vi "Constructor.vi"(8 "error in (no error)":errorcluster, 10 "lines":tag, 11 "Solenoid Valve in":refnum<class "Solenoid Valve.lvclass">) -> (0 "error out":errorcluster, 3 "Solenoid Valve out":refnum<class "Solenoid Valve.lvclass">)   [LabVIEW 2011, in "Solenoid Valve.lvclass"]
uses:
  Solenoid Valve.lvclass
  Solenoid Valve.lvclass/Solenoid Valve.ctl
  <vilib>/DAQmx/write.llb/DAQmx Write (Digital Bool 1Line 1Point).vi
  <vilib>/DAQmx/create/channels.llb/DAQmx Create Channel (DO-Digital Output).vi
  <vilib>/DAQmx/miscellaneous.llb/DAQmx Fill In Error Info.vi
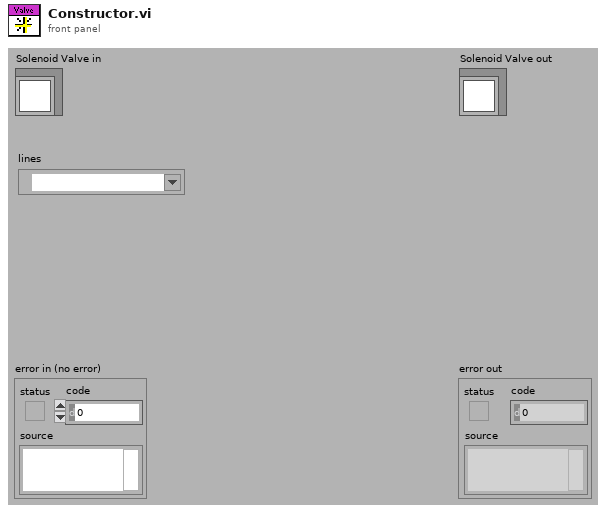
[diagram p1: front panel]
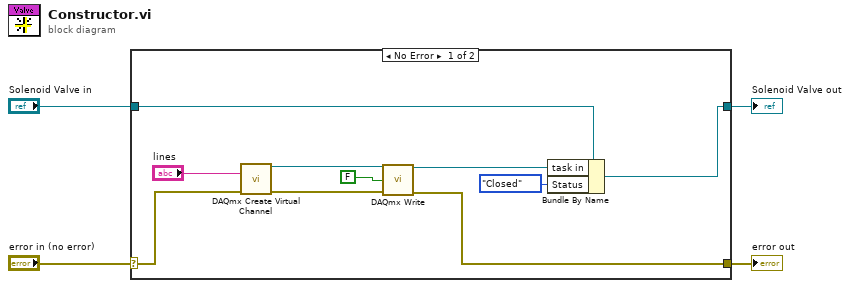
[diagram p0: block diagram]
diagram:
  n1 = case shown="No Error" "error in (no error)" {
    selector: "error in (no error)" -> [w8 w16]
    tunnel: [w6 w16] -> w3
    tunnel: [w9 w15] -> w1
    tunnel: "Solenoid Valve in" -> [w11 w15]
    frame No Error {
      n2 = call-poly <vilib>:"DAQmx Create Virtual Channel.vi"("lines"="lines", "error in"=w8) -> ("task out"=w13:refnum<k21>, "error out"=w7:errorcluster)  [unwired: 12 in]
      n3 = call-poly <vilib>:"DAQmx Write.vi"("task/channels in"=w13, "data"=FALSE, "error in"=w7) -> ("task out"=w10:refnum<k21>, "error out"=w6:errorcluster)  [unwired: 10 in, 1 out]
      n4 = Bundle By Name(cluster=w11, "task in"=w10, "Status"=enum16{"Closed", "Open"}."Closed") -> (w9:refnum<class "Solenoid Valve.lvclass">)
    }
    frame Error {
    }
  }
  "error out" <- w3
  "Solenoid Valve out" <- w1
